vi "06c-arrays.vi"() -> ()   [LabVIEW 2018, in "LV-0mq-Julia_roundtrip-lib.lvlib"]
uses:
  LV-0mq-Julia_roundtrip-lib.lvlib
  Server or client state.ctl
  statistics.ctl
  Commands.ctl
  ZMQ timeouts.ctl
  0d29fc62-3d1d-4713-a954-9c9e873b3633.vi
  aea790a6-a42b-4eb0-905f-734239196901.vi
  72a46192-383e-4ee5-9465-71670922b82a.vi
  ef5408d4-6538-41d1-b296-fda05a71e4b0.vi
  b8d67b76-17b0-4ad8-b521-2f6549c52c10.vi
  e4efb182-1b04-4d49-96a3-1defebd055ea.vi
  ef458cb0-9ca2-4aa9-bd1e-ad103f8bb0c0.vi
  9df197b6-2616-4b86-abf4-a70e9215d122.vi
  28751878-cf8c-4743-a8b0-c60d78ce5b36.vi
  c328879f-33e1-4261-a6aa-c93c9ebac265.vi
  0d29fc62-3d1d-4713-a954-9c9e873b3633.vi/8ee49078-a04b-40cf-aceb-de90d52f19ef.vi
  aea790a6-a42b-4eb0-905f-734239196901.vi/353007a7-a356-474a-8eac-0d4386ef6058.vi
  72a46192-383e-4ee5-9465-71670922b82a.vi/ea2ca31c-a649-493c-8d06-3a8000b732b1.vi
  ef5408d4-6538-41d1-b296-fda05a71e4b0.vi/365813fc-9c19-4b31-a490-477dd90e6dd4.vi
  b8d67b76-17b0-4ad8-b521-2f6549c52c10.vi/7972b5ea-775d-4b37-89ba-aaca190de37a.vi
  e4efb182-1b04-4d49-96a3-1defebd055ea.vi/f67e9a7a-314b-4767-8e61-05416f28844a.vi
  e4efb182-1b04-4d49-96a3-1defebd055ea.vi/dad3c3ea-dc05-4971-94cf-d4795e780bf2.vi
  ef458cb0-9ca2-4aa9-bd1e-ad103f8bb0c0.vi/e8b90c0a-49a5-4093-b01b-c91da666bc06.vi
  9df197b6-2616-4b86-abf4-a70e9215d122.vi/3b3d9898-3907-4a71-916f-494130455110.vi
  28751878-cf8c-4743-a8b0-c60d78ce5b36.vi/3538928f-68b5-407e-942c-941291388321.vi
  c328879f-33e1-4261-a6aa-c93c9ebac265.vi/f47398fc-33b4-40f0-b8b3-8fb77e1f33fa.vi
  c328879f-33e1-4261-a6aa-c93c9ebac265.vi/961c45df-4515-43ad-b13c-15194131653f.vi
  72a46192-383e-4ee5-9465-71670922b82a.vi/ea2ca31c-a649-493c-8d06-3a8000b732b1.vi/4cda02a8-52b1-4797-9517-7736628fdc16.vi
  ef5408d4-6538-41d1-b296-fda05a71e4b0.vi/365813fc-9c19-4b31-a490-477dd90e6dd4.vi/c1bf83d8-4e50-4008-8373-782bae7d23a9.vi
  b8d67b76-17b0-4ad8-b521-2f6549c52c10.vi/7972b5ea-775d-4b37-89ba-aaca190de37a.vi/b25fc983-96dc-447d-82d8-162e37917a7f.vi
  b8d67b76-17b0-4ad8-b521-2f6549c52c10.vi/7972b5ea-775d-4b37-89ba-aaca190de37a.vi/3b720f21-803d-4a5f-818a-21a8e23e7bcd.vi
  b8d67b76-17b0-4ad8-b521-2f6549c52c10.vi/7972b5ea-775d-4b37-89ba-aaca190de37a.vi/e4395531-fc01-469f-b52e-7d6a1a2ff01c.vi
  e4efb182-1b04-4d49-96a3-1defebd055ea.vi/f67e9a7a-314b-4767-8e61-05416f28844a.vi/e860bdc9-9a6c-469b-a66b-1958d74c50f1.vi
  e4efb182-1b04-4d49-96a3-1defebd055ea.vi/f67e9a7a-314b-4767-8e61-05416f28844a.vi/4207b333-fb15-4c1c-ad1e-079bdcf1ed8e.vi
  9df197b6-2616-4b86-abf4-a70e9215d122.vi/3b3d9898-3907-4a71-916f-494130455110.vi/62e7ec98-c1ae-43c0-9f88-97112e5a4bb1.vi
  28751878-cf8c-4743-a8b0-c60d78ce5b36.vi/3538928f-68b5-407e-942c-941291388321.vi/830d3731-fe09-489c-8b6c-b12cfa6834e1.vi
  28751878-cf8c-4743-a8b0-c60d78ce5b36.vi/3538928f-68b5-407e-942c-941291388321.vi/85016cd6-3f02-4459-bf42-5915eb86a1e8.vi
  28751878-cf8c-4743-a8b0-c60d78ce5b36.vi/3538928f-68b5-407e-942c-941291388321.vi/ab16f215-63e4-4edc-aa12-c714cc51aa51.vi
  c328879f-33e1-4261-a6aa-c93c9ebac265.vi/f47398fc-33b4-40f0-b8b3-8fb77e1f33fa.vi/8efd1eeb-438d-43b0-8ba8-3107802f6827.vi
  c328879f-33e1-4261-a6aa-c93c9ebac265.vi/f47398fc-33b4-40f0-b8b3-8fb77e1f33fa.vi/fb215118-768d-4f6f-a1a8-ea7aac2ddd2f.vi
  72a46192-383e-4ee5-9465-71670922b82a.vi/ea2ca31c-a649-493c-8d06-3a8000b732b1.vi/4cda02a8-52b1-4797-9517-7736628fdc16.vi/f6bd3a2a-1504-4020-af9c-daf7937f7973.vi
  ef5408d4-6538-41d1-b296-fda05a71e4b0.vi/365813fc-9c19-4b31-a490-477dd90e6dd4.vi/c1bf83d8-4e50-4008-8373-782bae7d23a9.vi/fa26639b-d519-4ace-9d6a-dd3a988d1d0b.vi
  e4efb182-1b04-4d49-96a3-1defebd055ea.vi/f67e9a7a-314b-4767-8e61-05416f28844a.vi/e860bdc9-9a6c-469b-a66b-1958d74c50f1.vi/d31b27cf-298c-40e6-9590-a3de09aac7a2.vi
  9df197b6-2616-4b86-abf4-a70e9215d122.vi/3b3d9898-3907-4a71-916f-494130455110.vi/62e7ec98-c1ae-43c0-9f88-97112e5a4bb1.vi/af258aa4-6186-4a84-a905-c49851658aa9.vi
  c328879f-33e1-4261-a6aa-c93c9ebac265.vi/f47398fc-33b4-40f0-b8b3-8fb77e1f33fa.vi/8efd1eeb-438d-43b0-8ba8-3107802f6827.vi/03414bfb-35cf-4b69-a323-a8798f4fb1ac.vi
  check ID validity.vi
  bindata_descr to JSON.vi
  check cluster field names.vi
  concat JSON.vi
  build request.vi
  Parse server response.vi
  log jl exceptions.vi
  <vilib>/Utility/error.llb/Error Cluster From Error Code.vi
panel:
  out "Statistics 1":T1={"size "=0, "mean"=nan, "median"=nan, "min"=nan, "max"=nan} caption="Statistics (ms)" {"min" format="%#.1f"; "max" format="%#.1f"; "median" format="%.1f"; "mean" format="%.1f"}
  in  "max size 1":i32=20 caption="sample max"
  out "Statistics 2":T1={"size "=0, "mean"=nan, "median"=nan, "min"=nan, "max"=nan} caption="Statistics (ms)" {"min" format="%#.1f"; "max" format="%#.1f"; "median" format="%.1f"; "mean" format="%.1f"}
  in  "max size 2":i32=20 caption="sample max"
  out "error info 2":string
  out "Julia roundtrip time (ms) 2":dbl format="%#.3f"
  in  "N - arr size 2":u16=4
  out "Input Matrix (NxN)2":dbl[][](array[numeric])=[[1.0, 0.0, 5.0], [4.0, 2.0, 1.0], [2.0, 2.0, 3.0]] format="%#.4g"
  in  "paus2":bool
  out "current error 2":errorcluster
  out "error info 1":string
  out "Julia roundtrip time (ms) 1":dbl format="%#.3f"
  in  "N - arr size 1":u16=4
  out "Solution Vector":dbl[](array[numeric]) format="%.4f"
  out "Known Vector":dbl[](array[numeric])=[22.0, 14.0, 18.0] format="%#.4g"
  out "Input Matrix (NxN) 1":dbl[][](array[numeric])=[[1.0, 0.0, 5.0], [4.0, 2.0, 1.0], [2.0, 2.0, 3.0]] format="%#.4g"
  in  "paus1":bool
  out "current error 1":errorcluster
  out "Eigenvalues":cdb[](array[numeric]) format="%.2f"
  out "final error":errorcluster
  in  "stop":bool
  out "ZMQ timeout":bool
  out "Jl Server state":T2
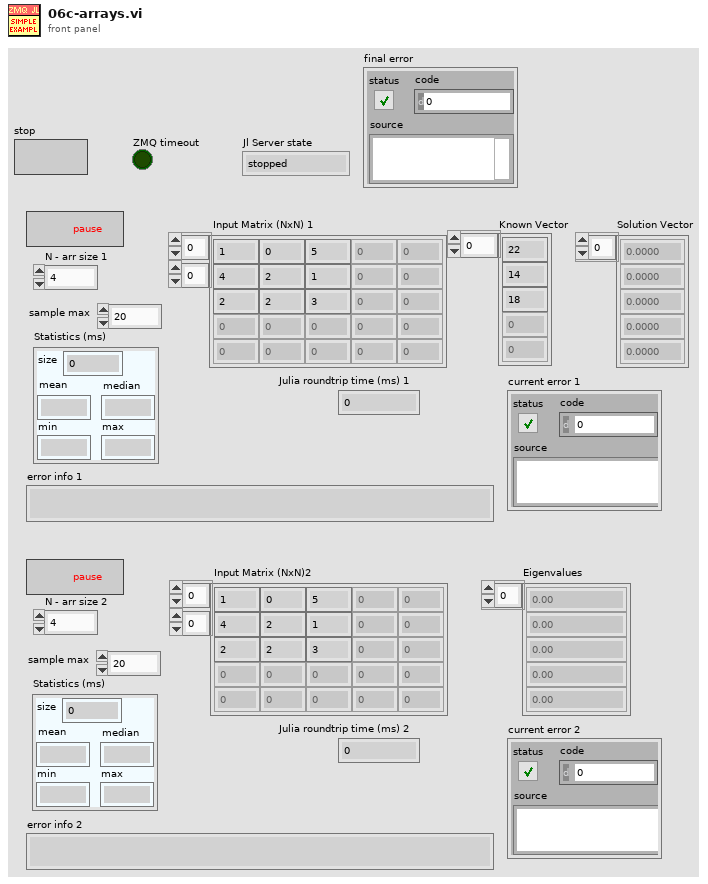
[diagram p1: front panel]
types:
  T1 = typedef "statistics.ctl" = cluster{"size ":u32, "mean":dbl, "median":dbl, "min":dbl, "max":dbl}
  T2 = typedef "LV-0mq-Julia_roundtrip-lib.lvlib/Server or client state.ctl" = enum16{"stopped", "running", "unknown"}
  T3 = typedef "LV-0mq-Julia_roundtrip-lib.lvlib/ZMQ timeouts.ctl" = cluster{"SNDTIMEO":i32, "RCVTIMEO":i32}
  T4 = typedef "LV-0mq-Julia_roundtrip-lib.lvlib/Commands.ctl" = enum16{"Start Jl-server & Init LV-client", "Send request & Get response ", "Stop Jl-server & Cleanup LV-client", "Cleanup LV-client", "Start Jl-server", "Stop Jl-server", "Init LV-Client", "Cleanup LV-Client", "(not allowed)", "Set LV Client state", "Set Jl Server state", "set ZMQ timeout", "read ZMQ timeout", "read-out state"}
  T5 = typedef "LV-0mq-Julia_roundtrip-lib.lvlib/Bindata&description.ctl" = cluster{"bindata_descr":T6[], "bindata":u8[]}
  T6 = typedef "LV-0mq-Julia_roundtrip-lib.lvlib/Bindata description.ctl" = cluster{"nofbytes":i32, "numtype":string, "start":i32, "arrdims":i32[], "kwarg_name":string, "category":string}
  T7 = typedef "LV-0mq-Julia_roundtrip-lib.lvlib/detailed error info.ctl" = cluster{"exception_or_info":string, "trace":T8[]}
  T8 = typedef "LV-0mq-Julia_roundtrip-lib.lvlib/StackFrame.ctl" = cluster{"frame_summary":string, "func":string, "linfo":string, "file":string, "line":i32, "pointer":u64, "from_c":bool, "inlined":bool}
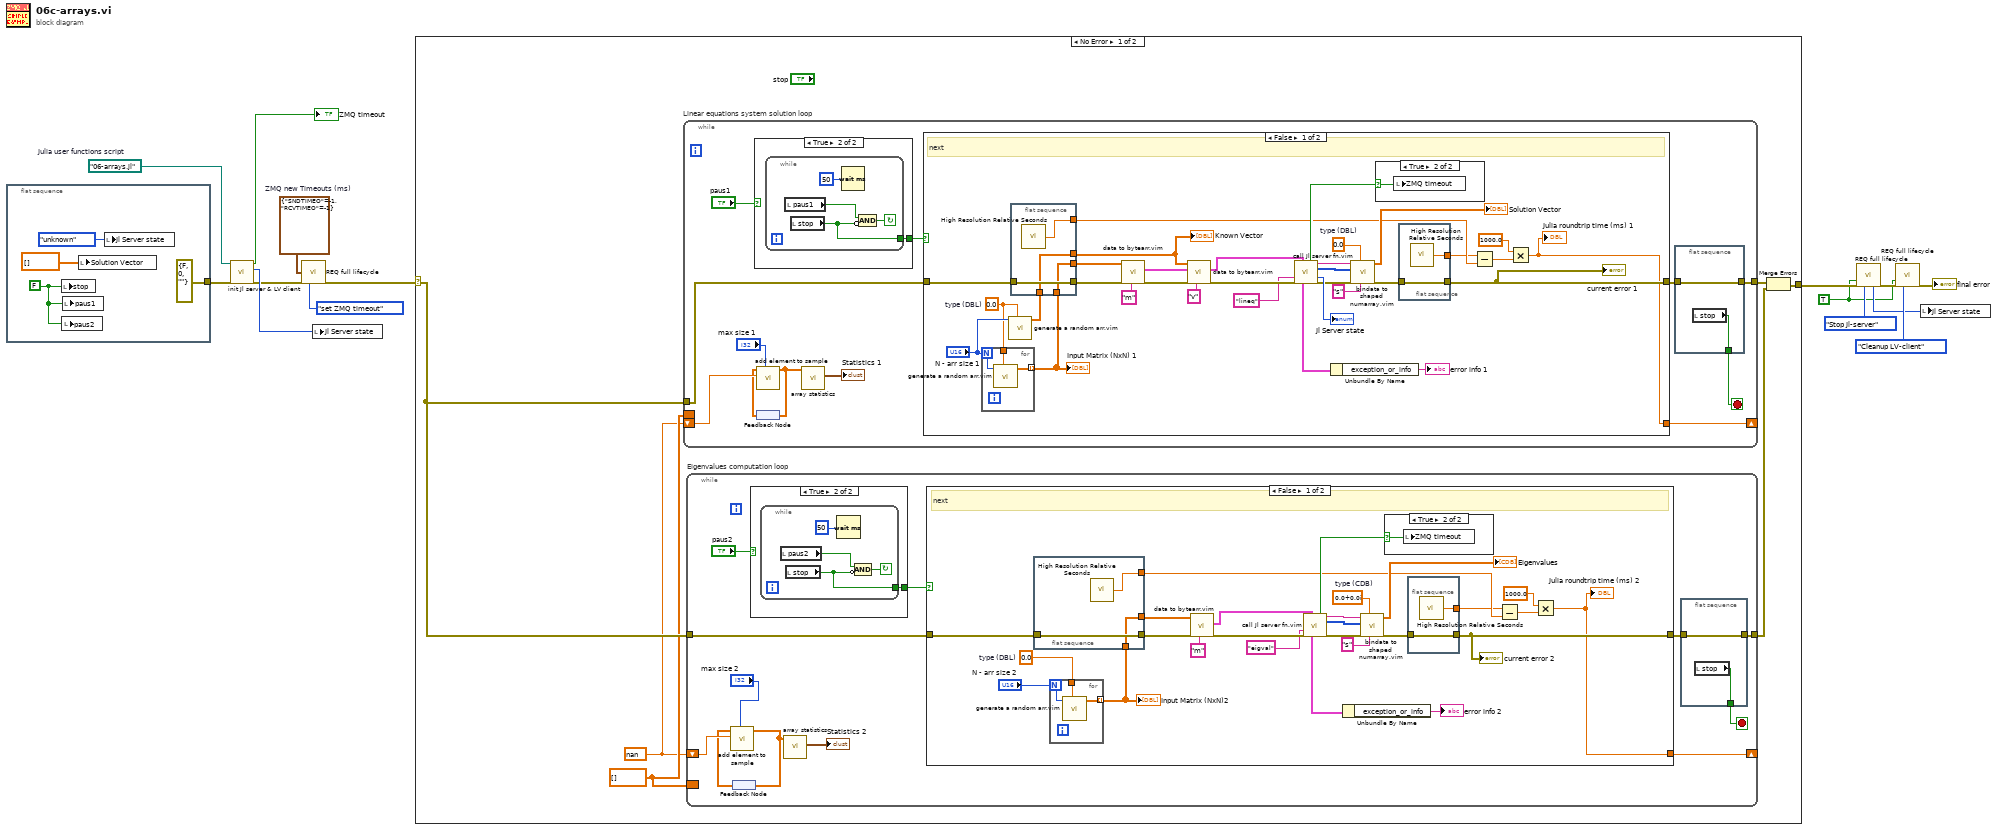
[diagram p0: block diagram]
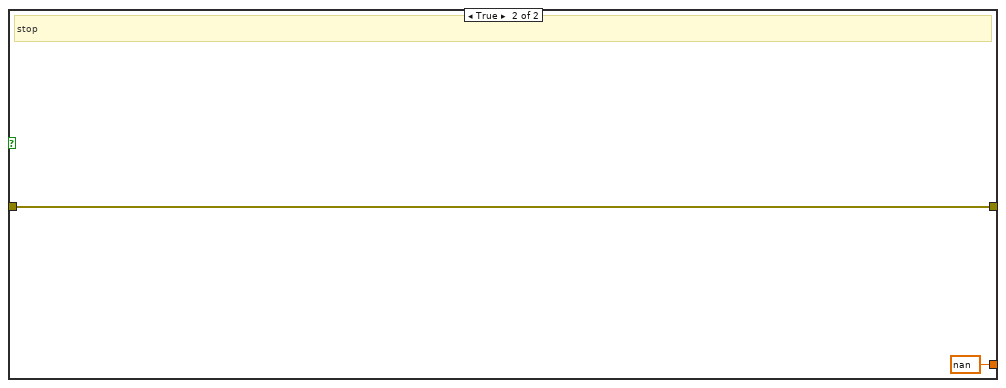
[diagram p4: hidden frame]
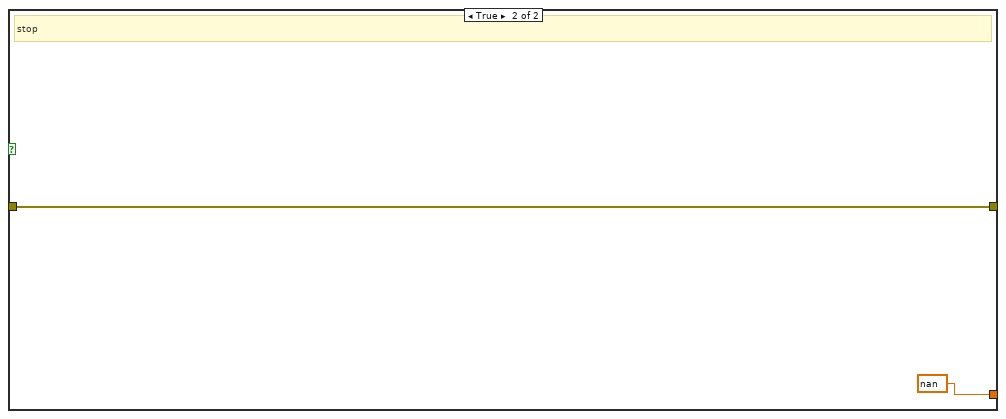
[diagram p7: hidden frame]
diagram:
  w6 = T3 {"SNDTIMEO"=-1, "RCVTIMEO"=-1}  # ZMQ new Timeouts (ms)
  w5 = path "06-arrays.jl"  # Julia user functions script
  w9 = TRUE ("Force command")
  n1 = flat-sequence {
    tunnel: [errorcluster {"status"=FALSE, "code"=0, "source"=""} ("error in (no error)")] -> w2
    frame #0 {
      w16 = FALSE ("stop")
      n2 = local write "stop"(w16) -> ()
      n3 = local write "paus2"(w16) -> ()
      n4 = local write "paus1"(w16) -> ()
      n5 = local write "Solution Vector"(dbl[] [] ("Server response")) -> ()
      n6 = local write "Jl Server state"(Server_or_client_state."unknown" ("Jl Server state out")) -> ()
    }
  }
  n7 = call "init Jl server & LV client.vi"("error in (no error)"=w2, "Julia user functions script"=w5) -> ("error out"=w1:errorcluster, "Jl Server state out"=w3:T2, "timeout?"=→"ZMQ timeout":bool)  [unwired: 7 in]
  n8 = call "REQ full lifecycle.vi"("ZMQ new Timeouts in"=w6, "error in"=w1, "command"=Commands."set ZMQ timeout") -> ("error out"=w8:errorcluster)  [unwired: 6 in, 6 out]
  n9 = local write "Jl Server state"(w3) -> ()
  n10 = case shown="No Error" w8 {
    selector: w8 -> [w22 w145]
    tunnel: [w24 w145] -> w15
    frame No Error {
      w21 = dbl[] []
      w20 = nan
      n11 = while "Linear equations system solution loop" {
        tunnel: w22 -> [w88]
        tunnel: [w92] -> w25
        shift-right: [w87] -> _
        shift-left: w20 -> [w86]
        border: w21 -> [_]
        stop <- w91 stop-if-true
        n12 = case shown="True" "paus1" {
          tunnel: [_ w94] -> w90
          frame False {
          }
          frame True {
            n13 = while {
              tunnel: [w95] -> w94
              stop <- w96 continue-if-true
              n14 = local read "paus1"() -> (w97:bool)
              n15 = local read "stop"() -> (w95:bool)
              n16 = Wait (ms)(milliseconds to wait=u32 50) -> ()  [unwired: 1 out]
              n17 = Compound Arithmetic op=AND(w97, invert w95) -> (w96:bool)
            }
          }
        }
        n18 = feedback #1() -> (w84:dbl[])
        n19 = call "add element to sample.vi"("sample size in"="max size 1", "element in"=w86, "Array in"=w84) -> ("Array out"=w85:dbl[])  [unwired: 8 in]
        n20 = feedback-in #1(w85) -> ()
        n21 = call "array statistics.vi"("Array in"=w85) -> ("Statistics (ms)"=→"Statistics 1":T1)  [unwired: 10 in]
        n22 = case shown="False" w90 {
          tunnel: [w102 w144] -> w93
          tunnel: w88 -> [w117 w144]
          tunnel: [w101 nan] -> w87
          frame False {
            w126 = 0.0  # type (DBL)
            w129 = 0.0  # type (DBL)
            # "next"
            n23 = for {
              N: "N - arr size 1" -> [w139]
              tunnel: [w141] -> w109 mode=indexing
              tunnel: w126 -> [w140]
              n24 = call "generate a random arr.vim"("type in"=w140, "arr size"=w139) -> ("float out"=w141:dbl[])  [unwired: 5 in, 4 out]
            }
            "Input Matrix (NxN) 1" <- w109
            n25 = call "generate a random arr.vim"("type in"=w126, "arr size"="N - arr size 1") -> ("float out"=w114:dbl[])  [unwired: 5 in, 4 out]
            n26 = flat-sequence {
              tunnel: [w138] -> w116
              tunnel: w117 -> [w138]
              tunnel: w109 -> [w137]
              tunnel: [w137] -> w115
              tunnel: [w136] -> w104
              tunnel: w114 -> [w136]
              tunnel: [w135] -> w112
              frame #0 {
                n27 = call <vilib>:"High Resolution Relative Seconds.vi"() -> ("relative seconds"=w135:dbl)
              }
            }
            n28 = call "data to bytearr.vim"("kwarg_name"="m", "error in (no error)"=w116, "data in"=w115) -> ("error out"=w132:errorcluster, "Bindata & descr out"=w131:T5)  [unwired: 6 in, 1 out]
            n29 = call "data to bytearr.vim"("kwarg_name"="v", "error in (no error)"=w132, "Bindata & descr in"=w131, "data in"=w104) -> ("error out"=w118:errorcluster, "Bindata & descr out"=w122:T5)  [unwired: 5 in, 1 out]
            n30 = call "call Jl server fn.vim"("Bindata & descr in"=w122, "fun2call"="lineq" ("Julia function name"), "error in (no error)"=w118) -> ("timeout?"=w121:bool, "JSON received"=w120:string, "binary data received"=w119:u8[], "Jl Server state out"=→"Jl Server state":T2, "detailed error info"=w106:T7, "error out"=w123:errorcluster)  [unwired: 6 in, 1 out]
            n31 = Unbundle By Name(w106) -> ("exception_or_info"=→"error info 1":string)
            n32 = call "bindata to shaped numarray.vim"("name"="s" ("kwarg_name"), "data type"=w129, "error in (no error)"=w123, "binary data"=w119, "JSON in"=w120) -> ("error out"=w113:errorcluster, "numarray 1D"=→"Solution Vector":dbl[])  [unwired: 3 in, 2 out]
            n33 = case shown="True" w121 {
              selector: w121 -> [_ w142]
              frame False {
              }
              frame True {
                n34 = local write "ZMQ timeout"(w142) -> ()
              }
            }
            n35 = flat-sequence {
              tunnel: [w134] -> w102
              tunnel: w113 -> [w134]
              tunnel: [w133] -> w108
              frame #0 {
                n36 = call <vilib>:"High Resolution Relative Seconds.vi"() -> ("relative seconds"=w133:dbl)
              }
            }
            n37 = Subtract(x=w108, y=w112) -> (x-y=w111:dbl)
            n38 = Multiply(x=1000.0, y=w111) -> (x*y=w101:dbl)
            "Julia roundtrip time (ms) 1" <- w101
            "current error 1" <- w102
            "Known Vector" <- w104
          }
          frame True {
            # "stop"
          }
        }
        n39 = flat-sequence {
          tunnel: w93 -> [w100]
          tunnel: [w100] -> w92
          tunnel: [w99] -> w91
          frame #0 {
            n40 = local read "stop"() -> (w99:bool)
          }
        }
      }
      n41 = while "Eigenvalues computation loop" {
        tunnel: w22 -> [w37]
        tunnel: [w35] -> w23
        shift-right: [w31] -> _
        shift-left: w20 -> [w30]
        border: w21 -> [_]
        stop <- w34 stop-if-true
        n42 = feedback #2() -> (w27:dbl[])
        n43 = call "add element to sample.vi"("sample size in"="max size 2", "element in"=w30, "Array in"=w27) -> ("Array out"=w29:dbl[])  [unwired: 8 in]
        n44 = feedback-in #2(w29) -> ()
        n45 = case shown="True" "paus2" {
          tunnel: [_ w38] -> w33
          frame False {
          }
          frame True {
            n46 = while {
              tunnel: [w39] -> w38
              stop <- w40 continue-if-true
              n47 = local read "paus2"() -> (w41:bool)
              n48 = local read "stop"() -> (w39:bool)
              n49 = Wait (ms)(milliseconds to wait=u32 50) -> ()  [unwired: 1 out]
              n50 = Compound Arithmetic op=AND(w41, invert w39) -> (w40:bool)
            }
          }
        }
        n51 = call "array statistics.vi"("Array in"=w29) -> ("Statistics (ms)"=→"Statistics 2":T1)  [unwired: 10 in]
        n52 = case shown="False" w33 {
          tunnel: [w48 w81] -> w36
          tunnel: w37 -> [w59 w81]
          tunnel: [w45 nan] -> w31
          frame False {
            w67 = 0.0  # type (DBL)
            w69 = cdb 0.0+0.0i  # type (CDB)
            # "next"
            n53 = flat-sequence {
              tunnel: [w75] -> w58
              tunnel: w59 -> [w75]
              tunnel: w49 -> [w74]
              tunnel: [w74] -> w57
              tunnel: [w73] -> w55
              frame #0 {
                n54 = call <vilib>:"High Resolution Relative Seconds.vi"() -> ("relative seconds"=w73:dbl)
              }
            }
            n55 = for {
              N: "N - arr size 2" -> [w76]
              tunnel: [w78] -> w49 mode=indexing
              tunnel: w67 -> [w77]
              n56 = call "generate a random arr.vim"("type in"=w77, "arr size"=w76) -> ("float out"=w78:dbl[])  [unwired: 5 in, 4 out]
            }
            "Input Matrix (NxN)2" <- w49
            n57 = call "data to bytearr.vim"("kwarg_name"="m", "error in (no error)"=w58, "data in"=w57) -> ("error out"=w60:errorcluster, "Bindata & descr out"=w64:T5)  [unwired: 6 in, 1 out]
            n58 = call "call Jl server fn.vim"("Bindata & descr in"=w64, "fun2call"="eigval" ("Julia function name"), "error in (no error)"=w60) -> ("timeout?"=w63:bool, "JSON received"=w62:string, "binary data received"=w61:u8[], "detailed error info"=w50:T7, "error out"=w65:errorcluster)  [unwired: 6 in, 2 out]
            n59 = Unbundle By Name(w50) -> ("exception_or_info"=→"error info 2":string)
            n60 = call "bindata to shaped numarray.vim"("name"="s" ("kwarg_name"), "data type"=w69, "error in (no error)"=w65, "binary data"=w61, "JSON in"=w62) -> ("error out"=w56:errorcluster, "numarray 1D"=→"Eigenvalues":cdb[])  [unwired: 3 in, 2 out]
            n61 = case shown="True" w63 {
              selector: w63 -> [_ w79]
              frame False {
              }
              frame True {
                n62 = local write "ZMQ timeout"(w79) -> ()
              }
            }
            n63 = flat-sequence {
              tunnel: [w72] -> w48
              tunnel: w56 -> [w72]
              tunnel: [w71] -> w52
              frame #0 {
                n64 = call <vilib>:"High Resolution Relative Seconds.vi"() -> ("relative seconds"=w71:dbl)
              }
            }
            n65 = Subtract(x=w52, y=w55) -> (x-y=w54:dbl)
            n66 = Multiply(x=1000.0, y=w54) -> (x*y=w45:dbl)
            "Julia roundtrip time (ms) 2" <- w45
            "current error 2" <- w48
          }
          frame True {
            # "stop"
          }
        }
        n67 = flat-sequence {
          tunnel: w36 -> [w44]
          tunnel: [w44] -> w35
          tunnel: [w43] -> w34
          frame #0 {
            n68 = local read "stop"() -> (w43:bool)
          }
        }
      }
      n69 = Merge Errors(w25, w23) -> (w24:errorcluster)
    }
    frame Error {
    }
  }
  n70 = call "REQ full lifecycle.vi"("Force command"=w9, "error in"=w15, "command"=Commands."Stop Jl-server") -> ("Jl Server state out"=w10:T2, "error out"=w13:errorcluster)  [unwired: 6 in, 5 out]
  n71 = call "REQ full lifecycle.vi"("Force command"=w9, "error in"=w13, "command"=Commands."Cleanup LV-client") -> ("error out"=→"final error":errorcluster)  [unwired: 6 in, 6 out]
  n72 = local write "Jl Server state"(w10) -> ()
